vi "Get Chassis Slots.vi"(3 "ChassisType":T1) -> (1 "Num of Slots":i32)   [LabVIEW 2012]
uses:
  Controls/Chassis Type.ctl
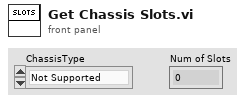
[diagram p1: front panel]
types:
  T1 = typedef "Chassis Type.ctl" = enum16{"Not Supported", "C Series 1-Slot", "C Series 4-Slot", "C Series 8-Slot", "PXI 8-Slot", "PXIe 18-Slot"}
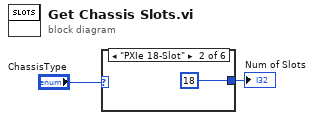
[diagram p0: block diagram]
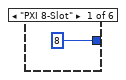
[diagram p2: hidden frame]
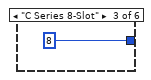
[diagram p3: hidden frame]
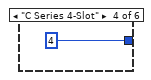
[diagram p4: hidden frame]
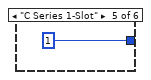
[diagram p5: hidden frame]
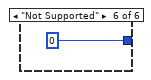
[diagram p6: hidden frame]
diagram:
  n1 = case shown="\"PXIe 18-Slot\"" "ChassisType" {
    tunnel: [8 ("dimension size") 18 ("dimension size") 8 ("dimension size") 4 ("dimension size") 1 ("dimension size") 0 ("dimension size")] -> w1
    frame "PXI 8-Slot" {
    }
    frame "PXIe 18-Slot" {
    }
    frame "C Series 8-Slot" {
    }
    frame "C Series 4-Slot" {
    }
    frame "C Series 1-Slot" {
    }
    frame "Not Supported" {
    }
  }
  "Num of Slots" <- w1
